vi "TraverseControl.vi"(0 "Mode":T6=enum."Read traverse position", 1 "Work in Tunnel Coordinates?":T3, 2 "Probe Support":T2=[{"Max"=15001.0, "Min"=12000.0}, {"Max"=1000.0, "Min"=-1000.0}, {"Max"=700.0, "Min"=0.0}] {"Min" format="%#.1f"; "Max" format="%#.1f"}, 3 "Model       Roll      Pitch       Yaw (deg)":sgl[](array[numeric]) format="%#.2f", 4 "Probe Volume":T2=[{"Max"=15.0, "Min"=-15.0}, {"Max"=250.0, "Min"=0.0}, {"Max"=15.0, "Min"=-15.0}] {"Min" format="%#.1f"; "Max" format="%#.1f"}, 5 "Position input XYZ":sgl[](array[numeric])=[0.0, 0.0, 0.0] format="%.2f", 6 "Route Checking?":bool, 7 "Entire Space":T2=[{"Max"=15001.0, "Min"=12000.0}, {"Max"=1000.0, "Min"=-1000.0}, {"Max"=700.0, "Min"=0.0}] {"Min" format="%#.1f"; "Max" format="%#.1f"}, 8 "Last Part of Move?":bool, 9 "Home":T1, 10 "Exclude Array":T4[](array[typedef]) {"Sizes"."Min" format="%#.1f"; "Sizes"."Max" format="%#.1f"}, 11 "Speed Factor":sgl=1.0 min=0.1 max=5 format="%.2f", 12 "Traverse Name":string, 13 "Backlash Compensation?":bool=TRUE) -> (14 "Position Output XYZ":sgl[](array[numeric]) format="%.2f", 17 "Moved?":bool, 19 "Error String":string)   [LabVIEW 2015]
uses:
  Anemometry/Anemometry Sub Vis/Gen Trav/Trav_mode.ctl
  Anemometry/Anemometry Sub Vis/Gen Trav/Route mapping/Exclude_cluster.ctl
  Anemometry/Anemometry Sub Vis/Gen Trav/Route mapping/Box_size.ctl
  Anemometry/Anemometry Sub Vis/Gen Trav/Route mapping/Exclusion_type.ctl
  Anemometry/Anemometry Sub Vis/Controls/Tunnel_Coordinates.ctl
  Anemometry/Anemometry Sub Vis/Controls/Home.ctl
  ~subVIs/GenericDriveCommand.ctl
  ADAM Client/Sub VIs/ADAM Controls/Update_scan_value.ctl
  Anemometry/Anemometry Sub Vis/Globals/Preference_global.vi
  Anemometry/Anemometry Sub Vis/Globals/Trav_pos_global.vi
  ~subVIs/DriveConfigGlobal.vi
panel:
  out "Config the same?":bool[](array[boolean])
  out "Server copy Location":path
  out "Position Steps":sgl[][](array[numeric]) format="%.2f"
  out "Log File":path
  out "Achieved Pos In Eng units of all channels":sgl[](array[numeric]) format="%.2f"
  out "Pulses Positon all channels":sgl[](array[numeric])
  out "Counters Reset?":bool
  # "X                Y                   Z"
  # "X                           Y                          Z"
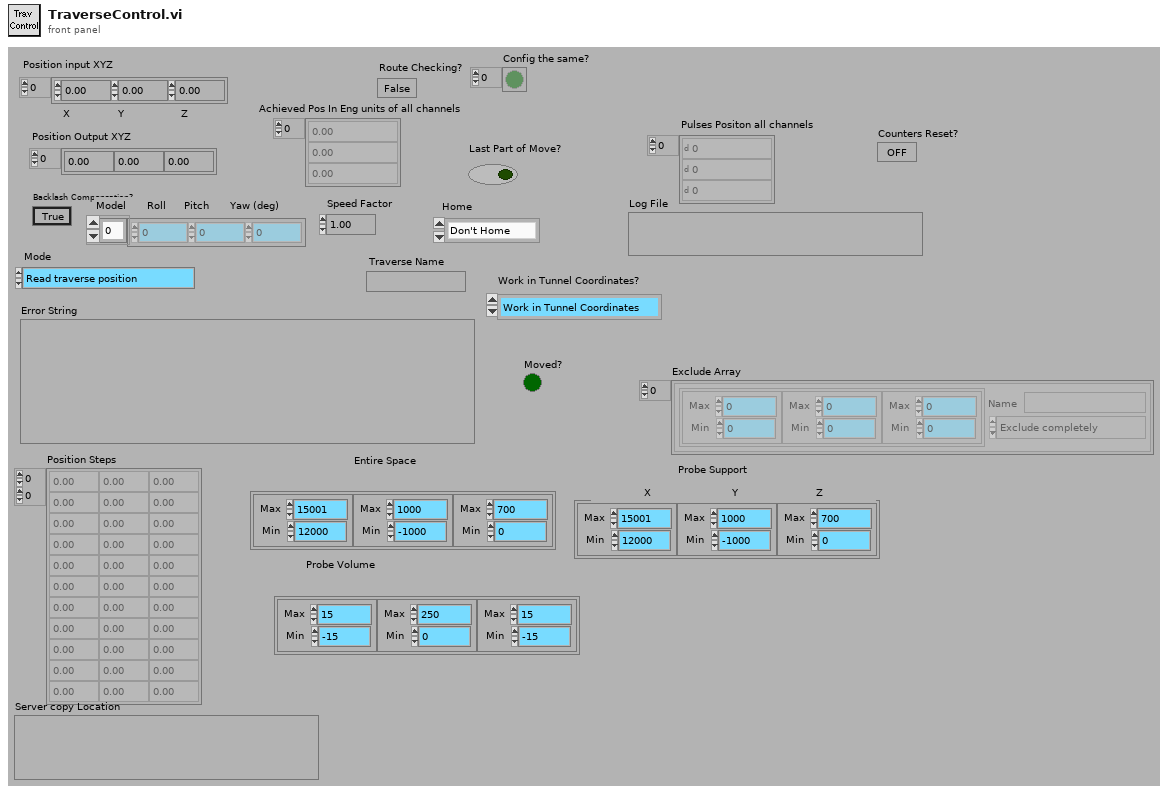
[diagram p1: front panel]
types:
  T1 = typedef "Home.ctl" = enum16{"Don't Home", "Home  +X", "Home  -X", "Home  +Y", "Home  -Y", "Home  +Z", "Home  -Z"}
  T2 = typedef "Box_size.ctl" = cluster{"Max":sgl, "Min":sgl}[]
  T3 = typedef "Tunnel_Coordinates.ctl" = enum16{"Work in Tunnel Coordinates", "Work in Model Coordinates"}
  T4 = typedef "Exclude_cluster.ctl" = cluster{"Sizes":T2, "Name":string, "Exclude Type":T5}
  T5 = typedef "Exclusion_type.ctl" = enum16{"Exclude completely", "Allow only vertical moves"}
  T6 = typedef "Trav_mode.ctl" = enum16{"Move traverse", "Read traverse position", "Teach Position"}
  T7 = typedef "GenericDriveCommand.ctl" = string
  T8 = enum16{"To Traverse Coordinates", "To User Coordinates"}
  T9 = typedef "Update_scan_value.ctl" = cluster{"Channel Name":string, "New Value":dbl}
  T10 = typedef "AxisConfigCluster.ctl" = cluster{"Channel Properties":T11, "Static Drive Configuration":T12}
  T11 = typedef "DriveProperties.ctl" = cluster{"Channel Name":string, "Vel. Default":sgl, "Acc. Default":sgl, "Vel. Max":sgl, "Vel. Min":sgl, "Acc. Max":sgl, "Acc. Min":sgl, "Pulses/unit":sgl, "Address":u8, "Pulse Offset":i32, "Pos Tolerance":sgl, "Pulses/rev":sgl, "Backlash/Eng units":sgl, "Current Pos":sgl, "Ch Status":enum16{"Active", "Offline", "Simulate"}, "Port Name":string, "Axis Transform mode":string, "Metadata Ch Name":string, "Type":string}
  T12 = typedef "DriveStaticConfig.ctl" = cluster{"Correction Gain % (CG)":u16, "Dead Band (DB)":i32, "Dead Band Window (DW)":i32, "Encoder Resolution (ER)":i32, "Step Mode  (FSB)":u16, "Position Maintenance (FSC)":u16, "Stop on Stall (FSD)":u16, "Activate OP1 on stall (FSE)":u16, "Stop on Trigger 3 (FSF)":u16, "OP2 in Deadband (FSG)":u16, "Stall Detect (FSH)":u16, "Limit Disable (LD)":u16, "Motor Resolution (MR)":enum16{"200", "400", "1000", "2000", "4000", "5000", "10000", "12800", "18000", "20000", "21600", "25000", "25400", "25600", "36000", "50000", "278528", "425984", "507904", "614400", "655360", "819200", "1024000"}, "Limit Switch Sense (OSA)":u16, "Home Position (OSB)":u16, "Home Switch Sense (OSC)":u16, "Encoder Z for Home (OSD)":u16, "Reference edge of Home (OSH)":u16, "RS232 Echo Control (SSA)":u16, "Buffer at Limit (SSG)":u16, "Buffer at Stop (SSH)":u16, "Indexer Mode  (FSA)":u16, "Type":string, "ConfigString":string, "De Power Motor":enum16{"TRUE", "FALSE"}}
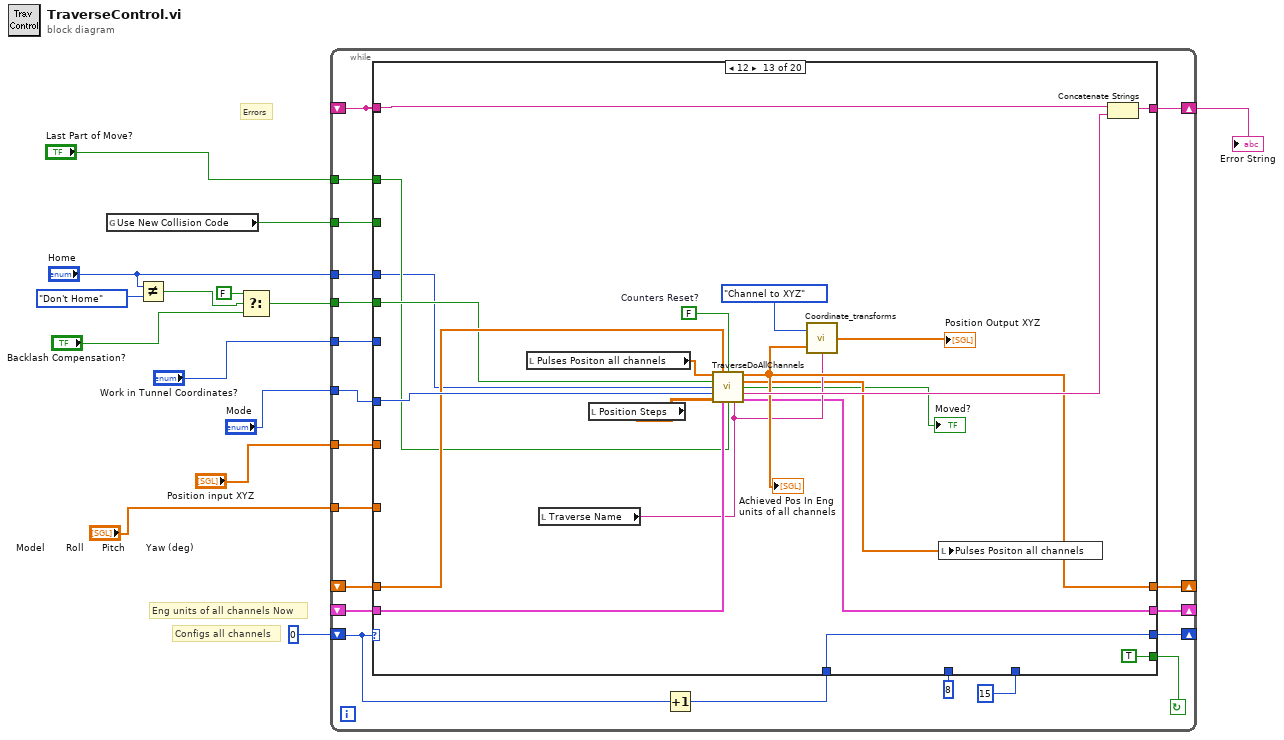
[diagram p0: block diagram]
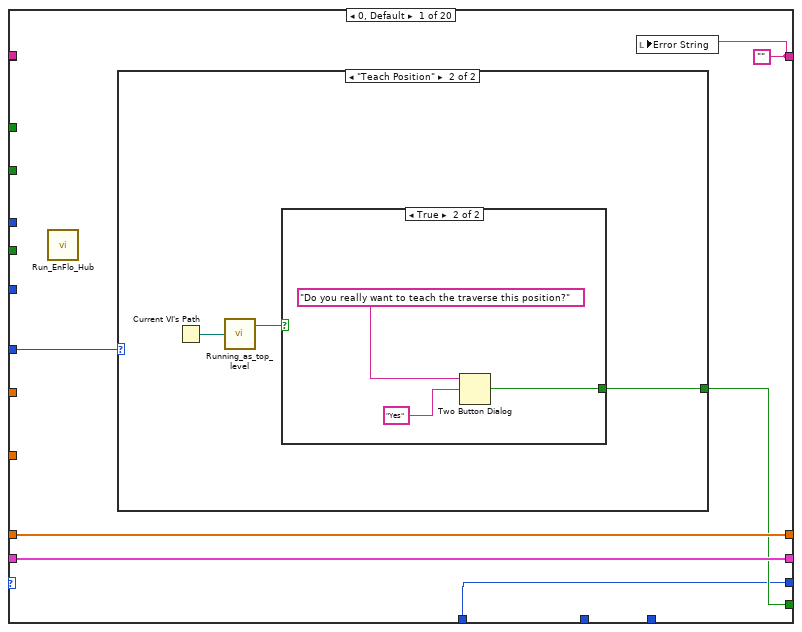
[diagram p2: hidden frame]
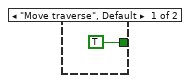
[diagram p3: hidden frame]
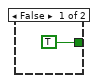
[diagram p4: hidden frame]
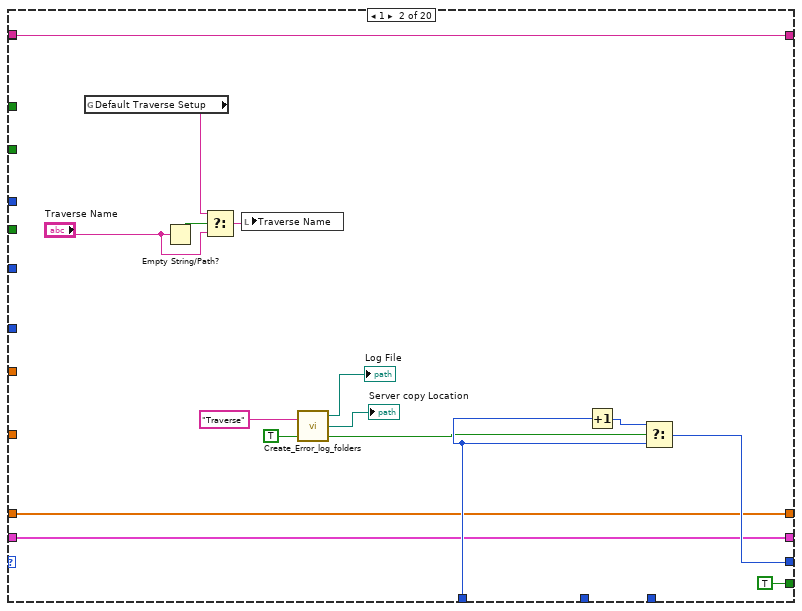
[diagram p5: hidden frame]
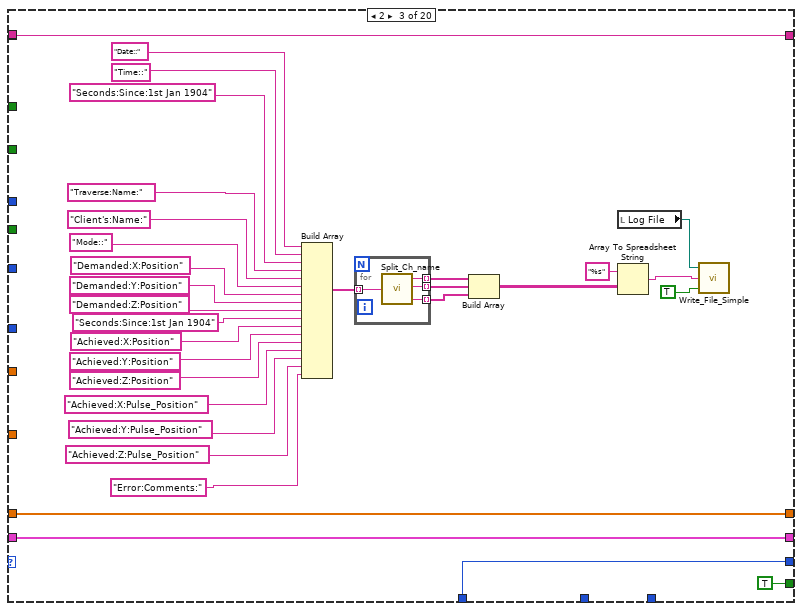
[diagram p6: hidden frame]
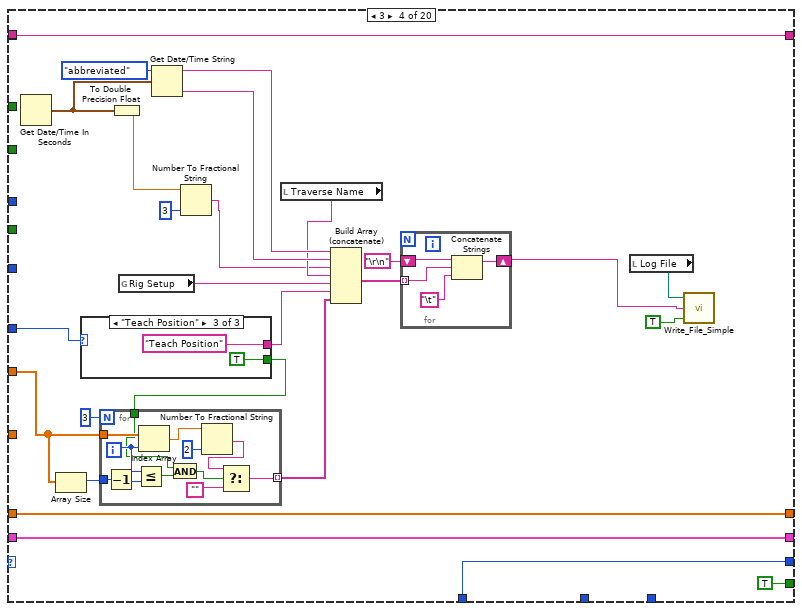
[diagram p7: hidden frame]
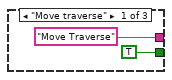
[diagram p8: hidden frame]
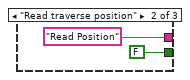
[diagram p9: hidden frame]
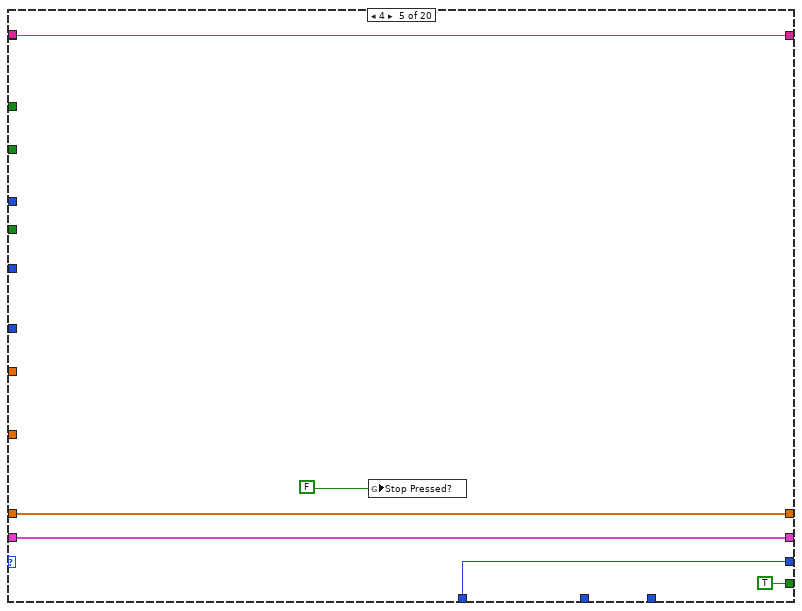
[diagram p10: hidden frame]
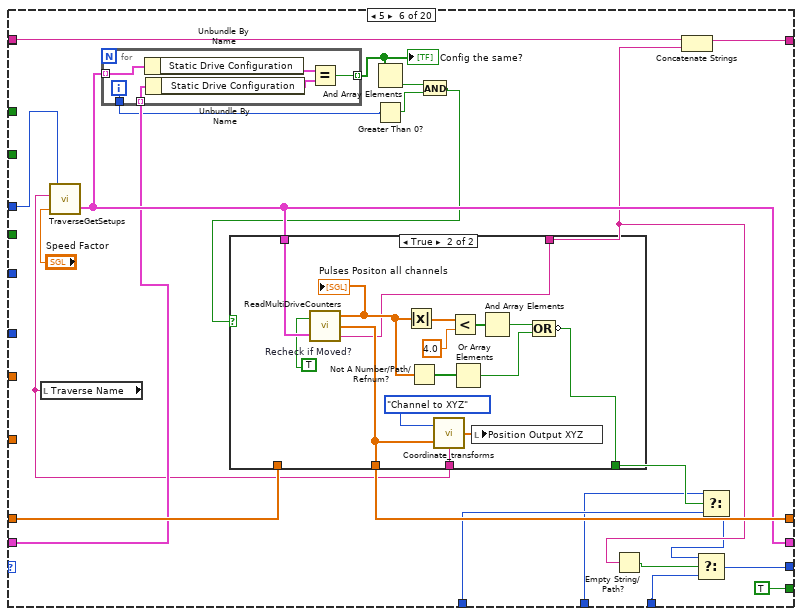
[diagram p11: hidden frame]
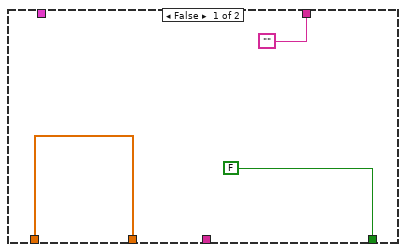
[diagram p12: hidden frame]
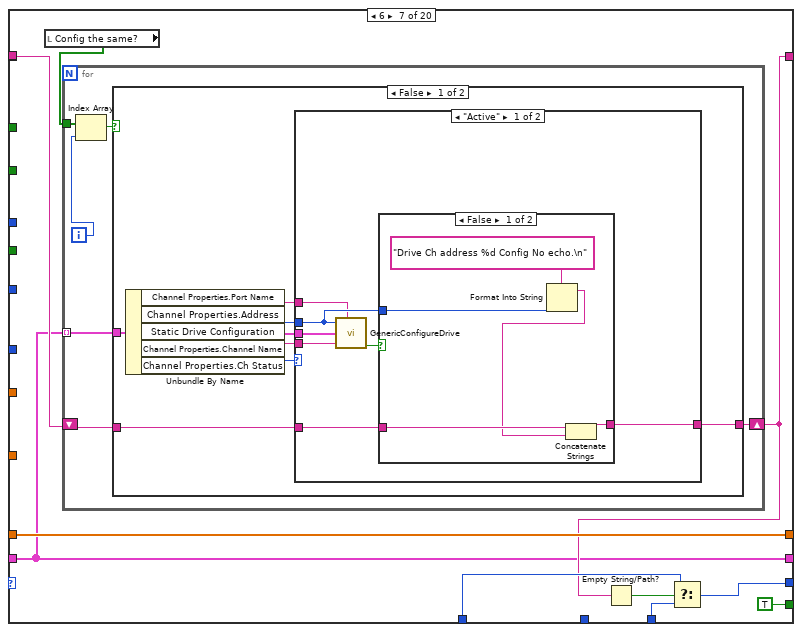
[diagram p13: hidden frame]
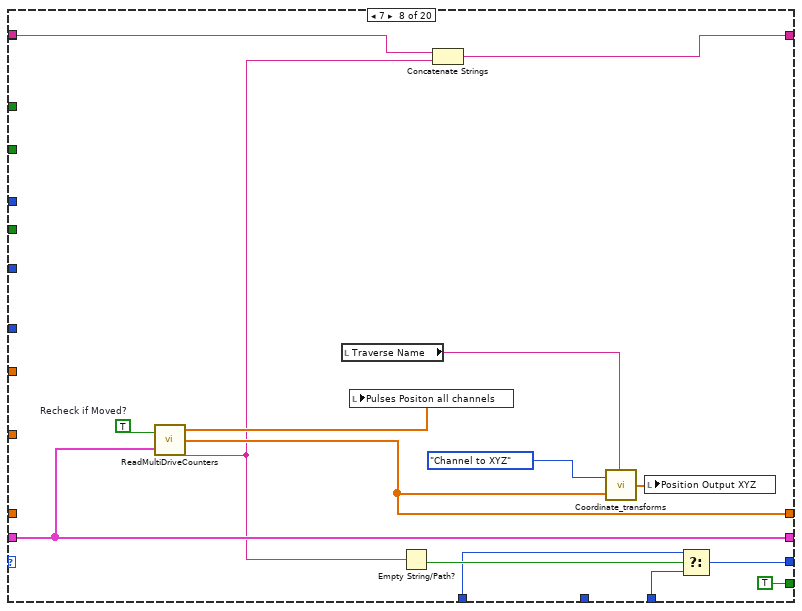
[diagram p17: hidden frame]
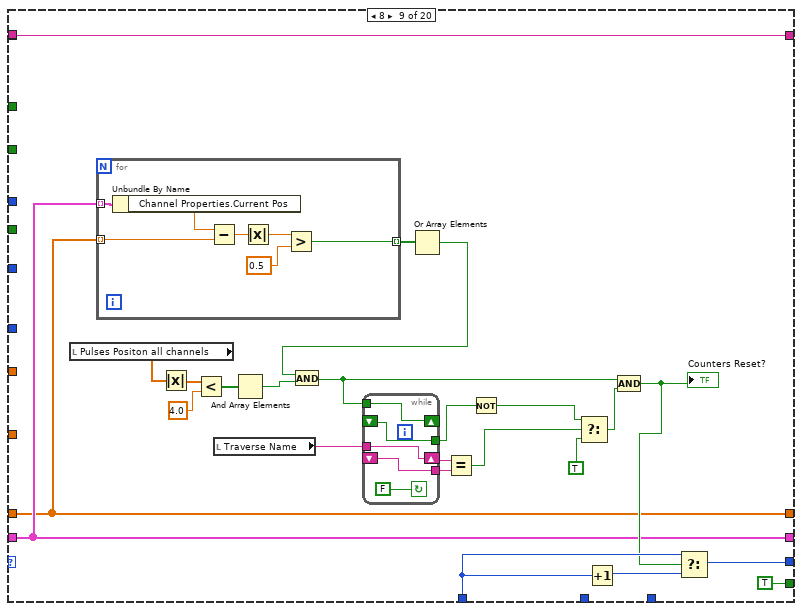
[diagram p18: hidden frame]
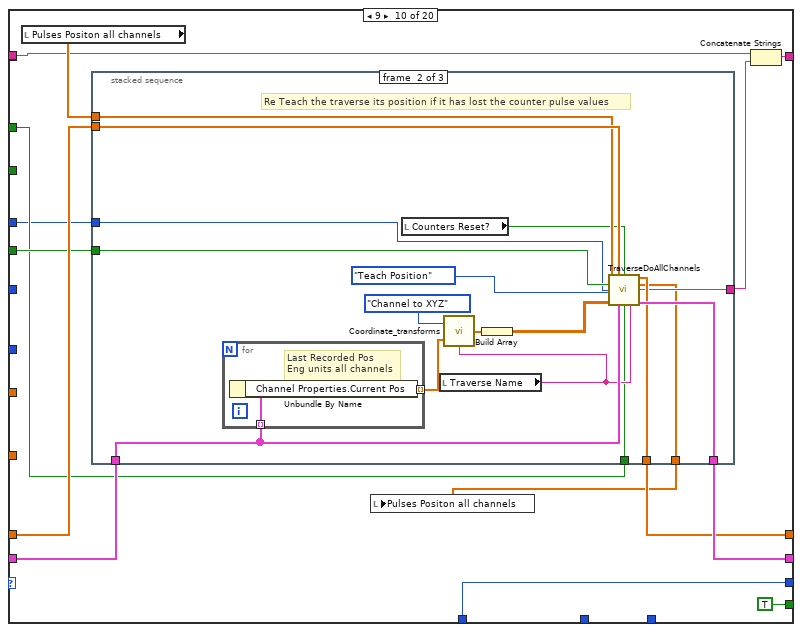
[diagram p19: hidden frame]
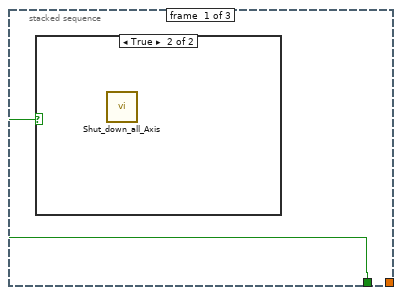
[diagram p20: hidden frame]
diagram:
  # "Errors"
  # "Eng units of all channels Now"
  # "Configs all channels"
  n1 = global read "Preference_global.vi" "Use New Collision Code"() -> (w1:bool)
  n2 = Not Equal?(x="Home", y=Home."Don't Home" ("Home")) -> (x != y?=w2:bool)
  n3 = Select(t=FALSE, s=w2, f="Backlash Compensation?") -> (s? t:f=w7:bool)
  n4 = while {
    tunnel: w7 -> [w21]
    tunnel: "Position input XYZ" -> [w25]
    shift-left: _ -> [w22]
    shift-right: [w26] -> w12
    shift-left: _ -> [w27]
    shift-right: [w28] -> _
    shift-left: _ -> [w16]
    shift-right: [w29] -> _
    shift-left: 0 -> [w32]
    shift-right: [w30] -> _
    tunnel: "Mode" -> [w34]
    tunnel: "Model       Roll      Pitch       Yaw (deg)" -> [w20]
    tunnel: "Work in Tunnel Coordinates?" -> [w19]
    tunnel: "Last Part of Move?" -> [w18]
    tunnel: "Home" -> [w17]
    tunnel: w1 -> [w15]
    stop <- w33 continue-if-true
    n5 = Increment(x=w32) -> (x+1=w31:i32)
    n6 = case shown="12" w32 {
      tunnel: w34 -> [w40 _ _ w118 _ _ _ _ _ _ w347 _ w432 w439 _ _ _ w507 _ w563]
      tunnel: [w37 TRUE ("T button?") TRUE ("T button?") TRUE ("T button?") TRUE TRUE ("T button?") TRUE ("T button?") TRUE ("T button?") TRUE TRUE TRUE ("T button?") TRUE ("T button?") TRUE TRUE TRUE ("T button?") TRUE ("T button?") TRUE ("T button?") w509 TRUE FALSE] -> w33
      tunnel: w31 -> [w36 w63 w75 w123 w148 w173 w207 w242 w274 w295 w346 w368 w423 w441 w457 w474 w502 w506 w541 w570]
      tunnel: [w36 w61 w75 w123 w148 w156 w206 w240 w272 w295 w345 w369 w423 w440 w457 w472 w502 w505 w541 w570] -> w30
      tunnel: [w38 w58 w77 w125 w150 w171 w202 w254 w269 w304 w343 w371 w416 w438 w459 w485 w504 w512 w539 w568] -> w29
      tunnel: w16 -> [w38 w58 w77 w125 w150 w170 w202 w254 w269 w303 w343 w371 w430 w438 w459 w485 w504 w512 w539 w568]
      tunnel: [w39 w59 w76 w124 w151 w176 w210 w249 w268 w300 w342 w361 w424 w444 w458 w484 w503 w513 w542 w571] -> w28
      tunnel: w27 -> [w39 w59 w76 w124 w151 w175 w210 _ w268 w301 w342 w361 w419 w444 w458 w484 w503 w513 w542 w571]
      tunnel: [w35 w57 w73 w115 w152 w161 w203 w245 w271 w297 w348 w364 w426 w442 w455 w476 w500 w508 w535 w564] -> w26
      tunnel: w22 -> [_ w57 w73 w115 w152 w162 w204 w246 w271 w299 w348 _ w427 w442 w455 w476 w500 w511 w537 w566]
      tunnel: w25 -> [_ _ _ w112 _ _ _ _ _ _ w341 w363 _ _ _ _ _ _ w533 _]
      tunnel: 15 ("f") -> [_ _ _ _ _ w157 w205 w241 _ _ _ w366 _ _ _ _ _ _ _ _]
      tunnel: 8 ("t") -> [_ _ _ _ _ w172 _ _ _ _ _ _ _ _ _ _ _ _ _ _]
      tunnel: w22 -> [_ _ _ _ _ _ _ _ _ _ _ w367 _ _ _ _ _ _ _ _]
      tunnel: w21 -> [_ _ _ _ _ _ _ _ _ w294 _ _ w418 _ _ _ _ _ _ _]
      tunnel: w20 -> [_ _ _ _ _ _ _ _ _ _ _ w358 _ _ _ _ _ _ w534 w561]
      tunnel: w19 -> [_ _ _ _ _ _ _ _ _ _ _ _ _ _ _ _ _ _ w531 w559]
      tunnel: w18 -> [_ _ _ _ _ _ _ _ _ w292 _ _ w414 w433 _ _ _ _ _ _]
      tunnel: w17 -> [_ _ _ _ _ w154 _ _ _ w291 _ _ w413 _ _ _ _ _ _ _]
      tunnel: w15 -> [_ _ _ _ _ _ _ _ _ _ _ w357 _ _ _ _ _ _ _ _]
      frame 0, Default {
        w35 = ""
        n7 = call "Run_EnFlo_Hub.vi"() -> ()  [unwired: 1 in, 7 out]
        n8 = case shown="\"Teach Position\"" w40 {
          tunnel: [TRUE ("T button?") w42] -> w37
          frame "Move traverse", Default {
          }
          frame "Teach Position" {
            n9 = Current VI's Path() -> (path=w44:path)
            n10 = call "Running_as_top_level.vi"("Vi path name"=w44) -> ("Top Level"=w43:bool)  [unwired: 1 out]
            n11 = case shown="True" w43 {
              tunnel: [TRUE ("T button?") w46] -> w42
              frame False {
              }
              frame True {
                n12 = Two Button Dialog(message="Do you really want to teach the traverse this position?", 2:"Yes" ("T button name (\"OK\")")) -> (T button?=w46:bool)  [unwired: 1 out]
              }
            }
          }
        }
        n13 = local write "Error String"(w35) -> ()
      }
      frame 1 {
        n14 = global read "Trav_pos_global.vi" "Default Traverse Setup"() -> (w54:string)
        n15 = Empty String/Path?(string/path="Traverse Name") -> (empty?=w52:bool)
        n16 = Select(t=w54, s=w52, f="Traverse Name") -> (s? t:f=w51:string)
        n17 = local write "Traverse Name"(w51) -> ()
        n18 = call "Create_Error_log_folders.vi"("Per Day Log File?"=TRUE, "Log Filename"="Traverse" ("Input Element")) -> ("exists?"=w55:bool, "Server copy Location"=→"Server copy Location":path, "Local Log File"=→"Log File":path)  [unwired: 1 in]
        n19 = Increment(x=w63) -> (x+1=w62:i32)
        n20 = Select(t=w62, s=w55, f=w63) -> (s? t:f=w61:i32)
      }
      frame 2 {
        n21 = Build Array("Date::", "Time::", "Seconds:Since:1st Jan 1904", "Traverse:Name:", "Client's:Name:", "Mode::", "Demanded:X:Position", "Demanded:Y:Position", "Demanded:Z:Position", "Seconds:Since:1st Jan 1904", "Achieved:X:Position", "Achieved:Y:Position", "Achieved:Z:Position", "Achieved:X:Pulse_Position", "Achieved:Y:Pulse_Position", "Achieved:Z:Pulse_Position", "Error:Comments:") -> (w80:string[])
        n22 = for {
          tunnel: w80 -> [w99] mode=indexing
          tunnel: [w98] -> w81 mode=indexing
          tunnel: [w97] -> w82 mode=indexing
          tunnel: [w96] -> w83 mode=indexing
          n23 = call "Split_Ch_name.vi"("Ch name"=w99) -> ("Top level"=w98:string, "Middle"=w97:string, "Low level"=w96:string)
        }
        n24 = Build Array(w81, w82, w83) -> (w78:string[][])
        n25 = local read "Log File"() -> (w70:path)
        n26 = Array To Spreadsheet String(array=w78, 3:"%s" ("format string")) -> (spreadsheet string=w71:string)  [unwired: 1 out]
        n27 = call "Write_File_Simple.vi"("append to file? (new file:F)"=TRUE, "character string"=w71, "file path"=w70) -> ()  [unwired: 2 out]
      }
      frame 3 {
        n28 = Get Date/Time In Seconds() -> (seconds since 1Jan1904=w104:timestamp)
        n29 = Array Size(array=w112) -> (size(s)=w113:i32)
        n30 = case shown="\"Teach Position\"" w118 {
          tunnel: ["Move Traverse" "Read Position" "Teach Position"] -> w119
          tunnel: [TRUE FALSE TRUE] -> w109
          frame "Move traverse" {
          }
          frame "Read traverse position" {
          }
          frame "Teach Position" {
          }
        }
        n31 = for {
          N: 3 -> [_]
          tunnel: w112 -> [w137]
          tunnel: w113 -> [w134]
          tunnel: [w130] -> w110 mode=indexing
          tunnel: w109 -> [w126]
          i -> [w132]
          n32 = Decrement(x=w134) -> (x-1=w133:i32)
          n33 = Less Or Equal?(x=w132, y=w133) -> (x <= y?=w128:bool)
          n34 = Index Array(array=w137, index=w132) -> (element=w136:sgl)
          n35 = And(x=w126, y=w128) -> (x .and. y?=w127:bool)
          n36 = Number To Fractional String(number=w136, precision (6)=i16 2) -> (F-format string=w131:string)  [unwired: 2 out]
          n37 = Select(t=w131, s=w127, f="") -> (s? t:f=w130:string)
        }
        n38 = To Double Precision Float(number=w104) -> (double precision float=w103:dbl)
        n39 = global read "Preference_global.vi" "Rig Setup"() -> (w100:string)
        n40 = Get Date/Time String(date format (0)=enum16{"short", "long", "abbreviated"}."abbreviated", seconds (now)=w104) -> (date string=w121:string, time string=w120:string)  [unwired: 1 out]
        n41 = Number To Fractional String(number=w103, precision (6)=i16 3) -> (F-format string=w101:string)  [unwired: 2 out]
        n42 = local read "Traverse Name"() -> (w105:string)
        n43 = Build Array (concatenate)(w121, w120, w101, w105, w100, w119, w110) -> (w116:string[])
        n44 = for {
          shift-right: [w140] -> w106
          shift-left: "\r\n" -> [w141]
          tunnel: w116 -> [w139] mode=indexing
          n45 = Concatenate Strings(w141, w139, "\t") -> (w140:string)
        }
        n46 = local read "Log File"() -> (w107:path)
        n47 = call "Write_File_Simple.vi"("append to file? (new file:F)"=TRUE, "character string"=w106, "file path"=w107) -> ()  [unwired: 2 out]
      }
      frame 4 {
        n48 = global write "DriveConfigGlobal.vi" "Stop Pressed?"(FALSE) -> ()
      }
      frame 5 {
        n49 = local read "Traverse Name"() -> (w164:string)
        n50 = call "TraverseGetSetups.vi"("Speed Factor"="Speed Factor", "Traverse Name"=w164, "Home"=w154) -> ("Matched Configurations"=w171:T10[])  [unwired: 1 in]
        n51 = for {
          tunnel: w171 -> [w182] mode=indexing
          tunnel: w170 -> [w181] mode=indexing
          tunnel: [w178] -> w169 mode=indexing
          tunnel: [w177] -> w168
          i -> [w177]
          n52 = Unbundle By Name(w182) -> ("Static Drive Configuration"=w180:T12)
          n53 = Unbundle By Name(w181) -> ("Static Drive Configuration"=w179:T12)
          n54 = Equal?(x=w180, y=w179) -> (x = y?=w178:bool)
        }
        "Config the same?" <- w169
        n55 = And Array Elements(Boolean array=w169) -> (logical AND=w166:bool)
        n56 = Greater Than 0?(x=w168) -> (x > 0?=w167:bool)
        n57 = And(x=w166, y=w167) -> (x .and. y?=w165:bool)
        n58 = case shown="True" w165 {
          tunnel: w171 -> [_ w200]
          tunnel: [w185 w190] -> w176
          tunnel: w175 -> [w185 _]
          tunnel: [FALSE w192] -> w174
          tunnel: w164 -> [_ w188]
          tunnel: ["" w186] -> w160
          frame False {
          }
          frame True {
            w187 = TRUE  # Recheck if Moved?
            n59 = call "ReadMultiDriveCounters.vi"("Recheck if Moved?"=w187, "Matched Configurations"=w200) -> ("Pulses"=w195:sgl[], "Eng units"=w190:sgl[], "Error String"=w186:string)
            "Pulses Positon all channels" <- w195
            n60 = Absolute Value(x=w195) -> (abs(x)=w199:sgl[])
            n61 = Not A Number/Path/Refnum?(number/path/refnum=w195) -> (NaN/Path/Refnum?=w194:bool[])
            n62 = call "Coordinate_transforms.vi"("Traverse Name"=w188, "Input"=w190, "Mode"=enum16{"XYZ to Channel", "Channel to XYZ"}."Channel to XYZ") -> ("Output"=w189:sgl[])
            n63 = Less?(x=w199, y=sgl 4.0 ("Achieved Position")) -> (x < y?=w197:bool[])
            n64 = Or Array Elements(Boolean array=w194) -> (logical OR=w193:bool)
            n65 = local write "Position Output XYZ"(w189) -> ()
            n66 = And Array Elements(Boolean array=w197) -> (logical AND=w196:bool)
            n67 = Compound Arithmetic op=OR(w196, w193) -> (invert w192:bool)
          }
        }
        n68 = Empty String/Path?(string/path=w160) -> (empty?=w159:bool)
        n69 = Concatenate Strings(w162, w160) -> (w161:string)
        n70 = Select(t=w172, s=w174, f=w173) -> (s? t:f=w158:i32)
        n71 = Select(t=w158, s=w159, f=w157) -> (s? t:f=w156:i32)
      }
      frame 6 {
        n72 = local read "Config the same?"() -> (w201:bool[])
        n73 = for {
          tunnel: w202 -> [w216] mode=indexing
          shift-right: [w214] -> w203
          shift-left: w204 -> [w215]
          tunnel: w201 -> [w212]
          i -> [w213]
          n74 = Index Array(array=w212, index=w213) -> (element=w211:bool)
          n75 = case shown="False" w211 {
            tunnel: w216 -> [w224 _]
            tunnel: w215 -> [w218 w239]
            tunnel: [w217 w239] -> w214
            frame False {
              n76 = Unbundle By Name(w224) -> ("Channel Properties.Port Name"=w219:string, "Channel Properties.Address"=w223:u8, "Static Drive Configuration"=w222:T12, "Channel Properties.Channel Name"=w221:string, "Channel Properties.Ch Status"=w220:enum16{"Active", "Offline", "Simulate"})
              n77 = case shown="\"Active\"" w220 {
                tunnel: w223 -> [w229 _]
                tunnel: w222 -> [w231 _]
                tunnel: w221 -> [w230 _]
                tunnel: w219 -> [w228 _]
                tunnel: w218 -> [w226 w238]
                tunnel: [w225 w238] -> w217
                frame "Active" {
                  n78 = call "GenericConfigureDrive.vi"("Address"=w229, "Port Name"=w228, "Static Drive Configuration"=w231, "Channel Name"=w230) -> ("Good Echo"=w227:bool)  [unwired: 4 out]
                  n79 = case shown="False" w227 {
                    tunnel: w229 -> [w236 _]
                    tunnel: w226 -> [w234 w237]
                    tunnel: [w233 w237] -> w225
                    frame False {
                      n80 = Format Into String(format string="Drive Ch address %d Config No echo.\n" ("Format String"), w236) -> (resulting string=w232:string)  [unwired: 2 in, 1 out]
                      n81 = Concatenate Strings(w234, w232) -> (w233:string)
                    }
                    frame True {
                    }
                  }
                }
                frame "Offline", Default {
                }
              }
            }
            frame True {
            }
          }
        }
        n82 = Empty String/Path?(string/path=w203) -> (empty?=w208:bool)
        n83 = Select(t=w207, s=w208, f=w205) -> (s? t:f=w206:i32)
      }
      frame 7 {
        w247 = TRUE  # Recheck if Moved?
        n84 = call "ReadMultiDriveCounters.vi"("Recheck if Moved?"=w247, "Matched Configurations"=w254) -> ("Pulses"=w252:sgl[], "Eng units"=w249:sgl[], "Error String"=w243:string)
        n85 = local read "Traverse Name"() -> (w248:string)
        n86 = local write "Pulses Positon all channels"(w252) -> ()
        n87 = Empty String/Path?(string/path=w243) -> (empty?=w244:bool)
        n88 = Concatenate Strings(w246, w243) -> (w245:string)
        n89 = call "Coordinate_transforms.vi"("Traverse Name"=w248, "Input"=w249, "Mode"=enum16{"XYZ to Channel", "Channel to XYZ"}."Channel to XYZ") -> ("Output"=w250:sgl[])
        n90 = local write "Position Output XYZ"(w250) -> ()
        n91 = Select(t=w242, s=w244, f=w241) -> (s? t:f=w240:i32)
      }
      frame 8 {
        n92 = local read "Pulses Positon all channels"() -> (w263:sgl[])
        n93 = for {
          tunnel: w269 -> [w290] mode=indexing
          tunnel: w268 -> [w288] mode=indexing
          tunnel: [w284] -> w266 mode=indexing
          n94 = Unbundle By Name(w290) -> ("Channel Properties.Current Pos"=w289:sgl)
          n95 = Subtract(x=w289, y=w288) -> (x-y=w287:sgl)
          n96 = Absolute Value(x=w287) -> (abs(x)=w286:sgl)
          n97 = Greater?(x=w286, y=0.5) -> (0:w284:bool)
        }
        n98 = Absolute Value(x=w263) -> (abs(x)=w278:sgl[])
        n99 = Less?(x=w278, y=4.0 ("Achieved Position")) -> (x < y?=w276:bool[])
        n100 = local read "Traverse Name"() -> (w262:string)
        n101 = And Array Elements(Boolean array=w276) -> (logical AND=w267:bool)
        n102 = Or Array Elements(Boolean array=w266) -> (logical OR=w265:bool)
        n103 = And(x=w265, y=w267) -> (x .and. y?=w264:bool)
        n104 = while {
          tunnel: [w282] -> w256
          tunnel: w264 -> [w283]
          shift-left: _ -> [w282]
          shift-right: [w283] -> _
          shift-right: [w280] -> w261
          shift-left: _ -> [w279]
          tunnel: w262 -> [w280]
          tunnel: [w279] -> w260
          stop <- FALSE continue-if-true
        }
        n105 = Equal?(x=w261, y=w260) -> (x = y?=w259:bool)
        n106 = Not(x=w256) -> (.not. x?=w255:bool)
        n107 = Select(t=w255, s=w259, f=TRUE) -> (s? t:f=w258:bool)
        n108 = Increment(x=w274) -> (x+1=w273:i32)
        n109 = Compound Arithmetic op=AND(w264, w258) -> (w270:bool)
        "Counters Reset?" <- w270
        n110 = Select(t=w274, s=w270, f=w273) -> (s? t:f=w272:i32)
      }
      frame 9 {
        n111 = local read "Pulses Positon all channels"() -> (w302:sgl[])
        n112 = stacked-sequence {
          tunnel: w302 -> [_ w314 w325]
          tunnel: [_ w322 _] -> w304
          tunnel: w301 -> [_ w321 _]
          tunnel: [_ w320 _] -> w300
          tunnel: w303 -> [_ w316 w326]
          tunnel: [_ w319 _] -> w298
          tunnel: w294 -> [_ w310 _]
          tunnel: [_ w308 _] -> w293
          tunnel: w292 -> [w305 w307 _]
          tunnel: w291 -> [_ w306 _]
          frame #0 {
            n113 = case shown="True" w305 {
              frame False {
              }
              frame True {
                n114 = call "Shut_down_all_Axis.vi"() -> ()  [unwired: 1 out]
              }
            }
          }
          frame #1 {
            # "Re Teach the traverse its position if it has lost the counter pulse values"
            n115 = for {
              tunnel: [w324] -> w315 mode=indexing
              tunnel: w316 -> [w323] mode=indexing
              # "Last Recorded Pos\nEng units all channels"
              n116 = Unbundle By Name(w323) -> ("Channel Properties.Current Pos"=w324:sgl)
            }
            n117 = local read "Counters Reset?"() -> (w312:bool)
            n118 = local read "Traverse Name"() -> (w311:string)
            n119 = call "Coordinate_transforms.vi"("Traverse Name"=w311, "Input"=w315, "Mode"=enum16{"XYZ to Channel", "Channel to XYZ"}."Channel to XYZ") -> ("Output"=w317:sgl[])
            n120 = Build Array(w317) -> (w309:sgl[][])
            n121 = call "TraverseDoAllChannels.vi"("Current Pulses positions for all channels"=w314, "Current Pos In Eng units of all channels"=w321, "Counters Reset?"=w312, "Backlash Compensation?"=w310, "Home"=w306, "Mode"=Trav_mode."Teach Position", "Position Steps"=w309, "Matched Configurations all Channels In"=w316, "Last Part of Move?"=w307, "Traverse Name"=w311) -> ("Achieved Pos In Eng units of all channels"=w320:sgl[], "Current Pulses positions for all channels Out"=w308:sgl[], "Error String"=w319:string, "Matched Configurations Out"=w322:T10[])  [unwired: 1 in, 1 out]
          }
          frame #2 {
            n122 = for {
              tunnel: w326 -> [w333] mode=indexing
              tunnel: w325 -> [w332] mode=indexing
              n123 = Unbundle By Name(w333) -> ("Channel Properties.Ch Status"=w331:enum16{"Active", "Offline", "Simulate"}, "Channel Properties.Port Name"=w330:string, "Channel Properties.Type"=w329:string, "Channel Properties.Address"=w328:u8, "Channel Properties.Channel Name"=w327:string)
              n124 = case shown="\"Active\"" w331 {
                tunnel: w332 -> [w339 _]
                tunnel: w330 -> [w338 _]
                tunnel: w329 -> [w337 _]
                tunnel: w328 -> [w336 _]
                tunnel: w327 -> [w335 _]
                frame "Active" {
                  n125 = call "GenericDriveIO.vi"("GenericDriveCommand"=T7 "PositionSetTarget", "Channel Name"=w335, "Numeric Value"=w339, "Address"=w336, "Type"=w337, "Port Name"=w338) -> ()  [unwired: 1 in, 5 out]
                }
                frame "Offline", Default {
                }
              }
            }
          }
        }
        n126 = local write "Pulses Positon all channels"(w293) -> ()
        n127 = Concatenate Strings(w299, w298) -> (w297:string)
      }
      frame 10 {
        n128 = Build Array(w341) -> (w340:sgl[][])
        n129 = local write "Position Steps"(w340) -> ()
        n130 = case shown="\"Read traverse position\", Default" w347 {
          tunnel: w346 -> [w349 w356]
          tunnel: [w351 w355] -> w345
          frame "Move traverse" {
            n131 = Increment(x=w349) -> (x+1=w350:i32)
            n132 = case shown="True" "Route Checking?" {
              tunnel: [w353 w354] -> w351
              tunnel: w350 -> [w353 _]
              tunnel: w349 -> [_ w354]
              frame False {
              }
              frame True {
              }
            }
          }
          frame "Read traverse position", Default {
            n133 = Increment(x=w356) -> (x+1=w355:i32)
          }
        }
      }
      frame 11 {
        n134 = local read "Traverse Name"() -> (w362:string)
        n135 = case shown="False" w357 {
          tunnel: w363 -> [w388 w408]
          tunnel: w362 -> [w387 w406]
          tunnel: w361 -> [w386 w410]
          tunnel: [w383 w403] -> w360
          tunnel: [w382 w404] -> w359
          tunnel: w358 -> [w376 w407]
          frame False {
            w381 = 0.1  # Reduce by
            w385 = TRUE  # Full Check
            n136 = for {
              tunnel: "Probe Volume" -> [w398] mode=indexing
              tunnel: [w397] -> w380 mode=indexing
              tunnel: w381 -> [w392]
              n137 = Unbundle By Name(w398) -> ("Max"=w396:sgl, "Min"=w394:sgl)
              n138 = Subtract(x=w396, y=w392) -> (x-y=w395:dbl)
              n139 = Add(x=w392, y=w394) -> (x+y=w393:dbl)
              n140 = Bundle By Name(cluster=w398, "Max"=w395, "Min"=w393) -> (w397:cluster{"Max":sgl, "Min":sgl})
            }
            n141 = call "Coordinate_transforms.vi"("Traverse Name"=w387, "Input"=w386, "Mode"=enum16{"XYZ to Channel", "Channel to XYZ"}."Channel to XYZ") -> ("Output"=w378:sgl[])
            n142 = call "Coordinate_rotation.vi"("Roll-Pitch-Yaw"=w376, "Input Position"=w378, "Mode"=T8."To User Coordinates") -> ("Output Position"=w377:sgl[])  [unwired: 2 in, 1 out]
            n143 = call "Coordinate_rotation.vi"("Roll-Pitch-Yaw"=w376, "Input Position"=w388, "Mode"=T8."To User Coordinates") -> ("Output Position"=w390:sgl[])  [unwired: 2 in, 1 out]
            n144 = call "Check_Traverse_move.vi"("Current position"=w377, "Traverse Name"=w387, "Full Check"=w385, "New Position"=w390, "Model       Roll      Pitch       Yaw (deg)"=w376, "Probe Volume"=w380, "Entire Space"="Entire Space", "Exclude Array"="Exclude Array", "Probe Support"="Probe Support") -> ("Steps"=w384:sgl[][], "Error Comments"=w382:string)  [unwired: 5 out]
            n145 = for {
              tunnel: w384 -> [w401] mode=indexing
              tunnel: [w400] -> w383 mode=indexing
              tunnel: w376 -> [w399]
              n146 = call "Coordinate_rotation.vi"("Roll-Pitch-Yaw"=w399, "Input Position"=w401, "Mode"=T8."To Traverse Coordinates") -> ("Output Position"=w400:sgl[])  [unwired: 2 in, 1 out]
            }
          }
          frame True {
            w405 = TRUE  # Full Check
            n147 = call "Coordinate_transforms.vi"("Traverse Name"=w406, "Input"=w410, "Mode"=enum16{"XYZ to Channel", "Channel to XYZ"}."Channel to XYZ") -> ("Output"=w409:sgl[])
            n148 = call "Check_Traverse_move_PN.vi"("Current position"=w409, "Traverse Name"=w406, "Full Check"=w405, "New Position"=w408, "Model       Roll      Pitch       Yaw (deg)"=w407) -> ("Steps"=w403:sgl[][], "Error Comments"=w404:string)  [unwired: 8 in, 1 out]
          }
        }
        "Position Steps" <- w360
        n149 = Empty String/Path?(string/path=w359) -> (empty?=w365:bool)
        n150 = Select(t=w368, s=w365, f=w366) -> (s? t:f=w369:i32)
        n151 = Concatenate Strings(w367, w359) -> (w364:string)
      }
      frame 12 {
        w421 = FALSE  # Counters Reset?
        n152 = local read "Pulses Positon all channels"() -> (w431:sgl[])
        n153 = local read "Traverse Name"() -> (w420:string)
        n154 = local read "Position Steps"() -> (w417:sgl[][])
        n155 = call "TraverseDoAllChannels.vi"("Current Pulses positions for all channels"=w431, "Current Pos In Eng units of all channels"=w419, "Counters Reset?"=w421, "Backlash Compensation?"=w418, "Home"=w413, "Mode"=w432, "Position Steps"=w417, "Matched Configurations all Channels In"=w430, "Last Part of Move?"=w414, "Traverse Name"=w420) -> ("Achieved Pos In Eng units of all channels"=w424:sgl[], "Current Pulses positions for all channels Out"=w415:sgl[], "Moved?"=→"Moved?":bool, "Error String"=w425:string, "Matched Configurations Out"=w416:T10[])  [unwired: 1 in]
        "Achieved Pos In Eng units of all channels" <- w424
        n156 = call "Coordinate_transforms.vi"("Traverse Name"=w420, "Input"=w424, "Mode"=enum16{"XYZ to Channel", "Channel to XYZ"}."Channel to XYZ") -> ("Output"=→"Position Output XYZ":sgl[])
        n157 = local write "Pulses Positon all channels"(w415) -> ()
        n158 = Concatenate Strings(w427, w425) -> (w426:string)
      }
      frame 13 {
        n159 = local read "Position Output XYZ"() -> (w436:sgl[])
        n160 = case shown="\"Teach Position\"" w439 {
          tunnel: w436 -> [_ w453 _]
          frame "Move traverse" {
          }
          frame "Read traverse position" {
            n161 = local write "Position input XYZ"(w453) -> ()
          }
          frame "Teach Position" {
            n162 = local write "Mode"(Trav_mode."Teach Position" ("Mode")) -> ()
          }
        }
        n163 = for {
          tunnel: w438 -> [w452] mode=indexing
          tunnel: T9 {"Channel Name"="", "New Value"=0.0} ("Update Scan Value Cluster") -> [w451]
          tunnel: w436 -> [w449] mode=indexing
          tunnel: [w448] -> w434 mode=indexing if=w446
          n164 = Unbundle By Name(w452) -> ("Channel Properties.Metadata Ch Name"=w450:string)
          n165 = Empty String/Path?(string/path=w450) -> (empty?=w447:bool)
          n166 = Bundle By Name(cluster=w451, "Channel Name"=w450, "New Value"=w449) -> (w448:T9)
          n167 = Not(x=w447) -> (.not. x?=w446:bool)
        }
        n168 = global write "DriveConfigGlobal.vi" "Run Emergency stop loop"(FALSE ("Run Emergency stop loop")) -> ()
        n169 = Increment(x=w441) -> (x+1=w440:i32)
        n170 = Not(x=w433) -> (.not. x?=w435:bool)
        n171 = call "Update_Current_Value_client.vi"("Don't Bother with check?"=w435, "Update array in"=w434) -> ()
      }
      frame 14 {
      }
      frame 15 {
        n172 = local read "Pulses Positon all channels"() -> (w462:sgl[])
        n173 = local read "Position Output XYZ"() -> (w461:sgl[])
        n174 = Get Date/Time In Seconds() -> (seconds since 1Jan1904=w471:timestamp)
        n175 = To Double Precision Float(number=w471) -> (double precision float=w464:dbl)
        n176 = Number To Fractional String(number=w464, precision (6)=i16 3) -> (F-format string=w463:string)  [unwired: 2 out]
        n177 = call "Remove_unprintable_Char.vi"("Input String"=w476) -> ("Output String"=w477:string)
        n178 = Build Array (concatenate)(w461, w462) -> (w460:sgl[])
        n179 = Array Size(array=w460) -> (size(s)=w479:i32)
        n180 = for {
          N: 6 -> [_]
          tunnel: w460 -> [w499]
          tunnel: w479 -> [w496]
          tunnel: [w491] -> w478 mode=indexing
          i -> [w494]
          n181 = Decrement(x=w496) -> (x-1=w495:i32)
          n182 = Less Or Equal?(x=w494, y=w495) -> (x <= y?=w493:bool)
          n183 = Index Array(array=w499, index=w494) -> (element=w498:sgl)
          n184 = Number To Fractional String(number=w498, precision (6)=i16 2) -> (F-format string=w492:string)  [unwired: 2 out]
          n185 = Select(t=w492, s=w493, f="") -> (s? t:f=w491:string)
        }
        n186 = Build Array (concatenate)(w463, w478, w477) -> (w481:string[])
        n187 = local read "Route Checking?"() -> (w475:bool)
        n188 = for {
          shift-right: [w488] -> w468
          shift-left: "" -> [w489]
          tunnel: w481 -> [w487] mode=indexing
          n189 = Concatenate Strings(w489, w487, "\t") -> (w488:string)
        }
        n190 = Increment(x=w474) -> (x+1=w473:i32)
        n191 = local read "Log File"() -> (w469:path)
        n192 = local read "Server copy Location"() -> (w466:path)
        n193 = Select(t=w473, s=w475, f=w474) -> (s? t:f=w472:i32)
        n194 = call "Write_File_Simple.vi"("append to file? (new file:F)"=TRUE, "character string"=w468, "file path"=w469) -> ("file path Out"=w467:path)  [unwired: 1 out]
        n195 = call "Updated_File_Copy.vi"("Target Path"=w466, "Source Path"=w467) -> ()  [unwired: 2 out]
      }
      frame 16 {
      }
      frame 17 {
        n196 = local read "Position Output XYZ"() -> (w514:sgl[])
        n197 = local read "Counters Reset?"() -> (w515:bool)
        n198 = Index Array(array=w514, index=2) -> (element=w520:sgl)
        n199 = Index Array(array=w514, index=0) -> (element=w522:sgl)
        n200 = Index Array(array=w514, index=1) -> (element=w521:sgl)
        n201 = Format Into String(format string="X= %.2f\tY= %.2f\tZ= %.2f" ("Format String"), w522, w521, w520) -> (resulting string=w523:string)  [unwired: 2 in, 1 out]
        n202 = case shown="\"Read traverse position\"" w507 {
          tunnel: w506 -> [w527 w529]
          tunnel: [w527 w528] -> w505
          frame "Move traverse", Default {
          }
          frame "Read traverse position" {
            n203 = Increment(x=w529) -> (x+1=w528:i32)
          }
        }
        n204 = Select(t="\nThe traverse was probably powered down since the last move. Its position has now been retaught and now all should be well.", s=w515, f="") -> (s? t:f=w516:string)
        n205 = call "Write_out_serial_log.vi"("Header message"=w523) -> ()
        n206 = Concatenate Strings(w511, w516) -> (w508:string)
        n207 = Empty String/Path?(string/path=w508) -> (empty?=w510:bool)
        n208 = Not(x=w510) -> (.not. x?=w509:bool)
      }
      frame 18 {
        # "Add demanded position"
        n209 = case shown="\"Work in Model Coordinates\"" w531 {
          tunnel: w534 -> [_ w549]
          tunnel: w533 -> [w544 w548]
          tunnel: [w544 w546] -> w532
          tunnel: [" (Tunnel Coordinates)" " (Model Coordinates)"] -> w530
          frame "Work in Tunnel Coordinates" {
          }
          frame "Work in Model Coordinates" {
            n210 = call "Coordinate_rotation.vi"("Roll-Pitch-Yaw"=w549, "Input Position"=w548, "Mode"=T8."To User Coordinates") -> ("Output Position"=w546:sgl[])  [unwired: 2 in, 1 out]
          }
        }
        n211 = for {
          tunnel: w539 -> [w557] mode=indexing
          shift-right: [w552] -> w536
          shift-left: "\nDem Pos " -> [w555]
          tunnel: w532 -> [w550] mode=indexing
          n212 = Unbundle By Name(w557) -> ("Channel Properties.Channel Name"=w556:string)
          n213 = call "Split_Ch_name.vi"("Ch name"=w556) -> ("Low level"=w554:string)  [unwired: 2 out]
          n214 = Format Into String(format string="%s=%.1f, " ("Format String"), w554, w550) -> (resulting string=w551:string)  [unwired: 2 in, 1 out]
          n215 = Concatenate Strings(w555, w551) -> (w552:string)
        }
        n216 = Concatenate Strings(w537, w536, w530) -> (w535:string)
      }
      frame 19 {
        # "Add Achieved Position"
        n217 = local read "Position Output XYZ"() -> (w558:sgl[])
        n218 = case shown="\"Work in Model Coordinates\"" w559 {
          tunnel: w561 -> [_ w575]
          tunnel: [w572 w574] -> w560
          tunnel: w558 -> [w572 w573]
          frame "Work in Tunnel Coordinates" {
          }
          frame "Work in Model Coordinates" {
            n219 = call "Coordinate_rotation.vi"("Roll-Pitch-Yaw"=w575, "Input Position"=w573, "Mode"=T8."To User Coordinates") -> ("Output Position"=w574:sgl[])  [unwired: 2 in, 1 out]
          }
        }
        n220 = for {
          tunnel: w568 -> [w587] mode=indexing
          shift-right: [w582] -> w565
          shift-left: "\nAchieved Pos " -> [w585]
          tunnel: w560 -> [w580] mode=indexing
          n221 = Unbundle By Name(w587) -> ("Channel Properties.Channel Name"=w586:string)
          n222 = call "Split_Ch_name.vi"("Ch name"=w586) -> ("Low level"=w584:string)  [unwired: 2 out]
          n223 = Format Into String(format string="%s=%.1f, " ("Format String"), w584, w580) -> (resulting string=w581:string)  [unwired: 2 in, 1 out]
          n224 = Concatenate Strings(w585, w581) -> (w582:string)
        }
        n225 = case shown="\"Move traverse\"" w563 {
          tunnel: ["When requesting a move." "When reading position." "When teaching position."] -> w562
          frame "Move traverse" {
          }
          frame "Read traverse position" {
          }
          frame "Teach Position" {
          }
        }
        n226 = Concatenate Strings(w566, w565, w562) -> (w564:string)
      }
    }
  }
  "Error String" <- w12
